vi "genDOE.vi"(8 "error in (no error)":errorcluster, 11 "db_File":path=path "C:/Users/YuanYuan/Desktop/Labview Data/Database") -> (0 "error out":errorcluster, 3 "Array 2":T1(array[cluster]))   [LabVIEW 2014]
uses:
  <vilib>/addons/database/Connection.llb/DB Tools Open Connec (String).vi
  <vilib>/addons/database/NI_Database_API.lvlib
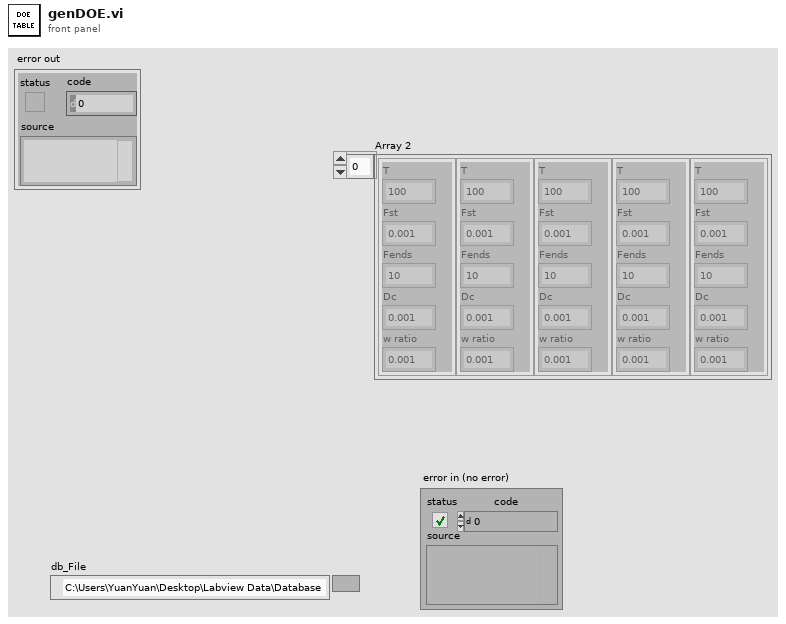
[diagram p1: front panel]
types:
  T1 = cluster{"T":dbl, "Fst":dbl, "Fends":dbl, "Dc":dbl, "w ratio":dbl}[]
  T2 = typedef "NI_Database_API.lvlib/Conn ObjectReference.ctl" = refnum<k1>
  T3 = cluster{"T":dbl, "Fst":dbl, "Fends":dbl, "Dc":dbl, "w ratio":dbl}
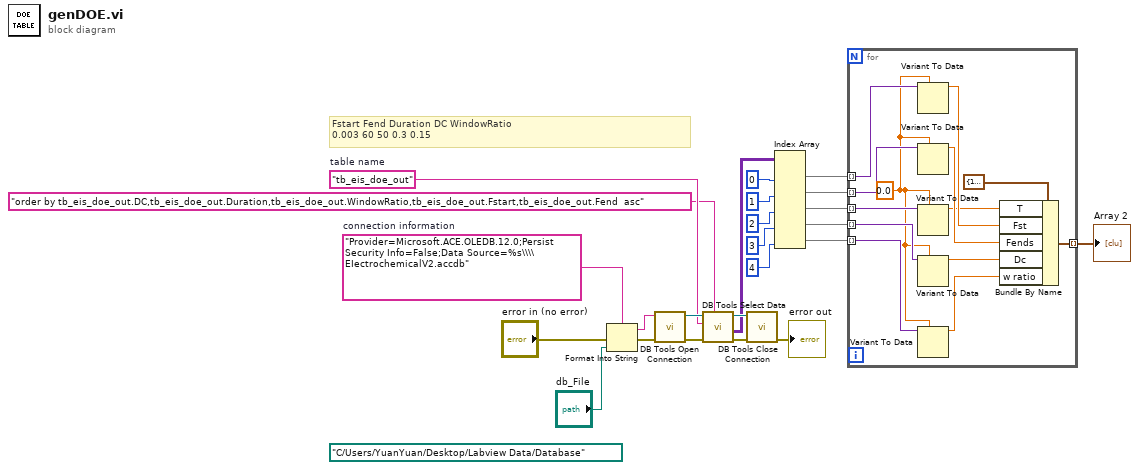
[diagram p0: block diagram]
diagram:
  (unwired) path "C:/Users/YuanYuan/Desktop/Labview Data/Database" ("path")
  w23 = "Provider=Microsoft.ACE.OLEDB.12.0;Persist Security Info=False;Data Source=%s\\\\EIectrochemicalV2.accdb"  # connection information
  w21 = "tb_eis_doe_out"  # table name
  # "Fstart\tFend\tDuration\tDC\tWindowRatio\n0.003\t60\t50\t0.3\t0.15"
  n1 = Format Into String(format string=w23, error in="error in (no error)", "db_File") -> (resulting string=w24:string, error out=w17:errorcluster)  [unwired: 1 in]
  n2 = call-poly <vilib>:"DB Tools Open Connection.vi"("error in (no error)"=w17, "connection information"=w24) -> ("error out"=w20:errorcluster, "connection reference"=w22:T2)  [unwired: 6 in]
  n3 = call <vilib>:"DB Tools Select Data.vi"("condition"="order by tb_eis_doe_out.DC,tb_eis_doe_out.Duration,tb_eis_doe_out.WindowRatio,tb_eis_doe_out.Fstart,tb_eis_doe_out.Fend  asc", "error in (no error)"=w20, "table"=w21, "connection reference"=w22) -> ("error out"=w15:errorcluster, "data"=w14:variant[][], "connection reference out"=w16:T2)  [unwired: 2 in]
  n4 = call <vilib>:"DB Tools Close Connection.vi"("error in (no error)"=w15, "connection reference"=w16) -> ("error out"=→"error out":errorcluster)  [unwired: 5 in]
  n5 = Index Array(array=w14, index (col) #1=0 ("disabled index (col)"), index (col) #2=1 ("index (col)"), index (col) #3=2 ("index (col)"), index (col) #4=3 ("index (col)"), index (col) #5=4 ("index (col)")) -> (element #1=w8:variant[], element #2=w7:variant[], element #3=w6:variant[], element #4=w5:variant[], element #5=w4:variant[])  [unwired: 5 in]
  n6 = for {
    tunnel: w8 -> [w36] mode=indexing
    tunnel: w7 -> [w34] mode=indexing
    tunnel: w6 -> [w32] mode=indexing
    tunnel: w5 -> [w30] mode=indexing
    tunnel: w4 -> [w27] mode=indexing
    tunnel: [w25] -> w3 mode=indexing
    w28 = 0.0 ("T")
    n7 = Variant To Data(type=w28, Variant=w36) -> (data=w35:dbl)  [unwired: 1 in, 1 out]
    n8 = Variant To Data(type=w28, Variant=w34) -> (data=w33:dbl)  [unwired: 1 in, 1 out]
    n9 = Variant To Data(type=w28, Variant=w32) -> (data=w31:dbl)  [unwired: 1 in, 1 out]
    n10 = Variant To Data(type=w28, Variant=w30) -> (data=w29:dbl)  [unwired: 1 in, 1 out]
    n11 = Variant To Data(type=w28, Variant=w27) -> (data=w26:dbl)  [unwired: 1 in, 1 out]
    n12 = Bundle By Name(cluster=T3 {"T"=150.0, "Fst"=0.001, "Fends"=10.0, "Dc"=0.0, "w ratio"=0.1} ("DOE parameters"), "T"=w31, "Fst"=w35, "Fends"=w33, "Dc"=w29, "w ratio"=w26) -> (w25:T3)
  }
  "Array 2" <- w3
